vi "killApplication.vi"(8 "error in (no error)":errorcluster, 11 "VGS_RemoteControlClient in":refnum<class "VGS_RemoteControlClient.lvclass">) -> (0 "error out":errorcluster, 3 "VGS_RemoteControlClient out":refnum<class "VGS_RemoteControlClient.lvclass">)   [LabVIEW 2022 SP3, in "LV_VGS.lvlib" / "VGS_RemoteControlClient.lvclass"]
doc: "<B>Kills an existing VGStudio (MAX) instance. </B>\n\nThis method kills a running VGStudio (MAX) instance process, using the respective RemoteHandle. The method is used to unconditionally cause an application instance process to exit.\n\nParameters\nhandle A valid handle to an application instance. \n\nEmit error RemoteControlServiceIsNotAvailableException if the remote control service doesn't run. \nEmit error GenericRemoteControlErrorException if an internal error occurs.\nEmit error InvalidRemoteHandleException if the remote handle is not valid."
uses:
  VGS_RemoteControlClient.lvclass
  VGS_RemoteControlClient.lvclass/VGS_RemoteControlClient.ctl
  C:/Users/Andrey/Desktop/hajo/LV_VGS/vgs_project.dll
  vgs_project.dll
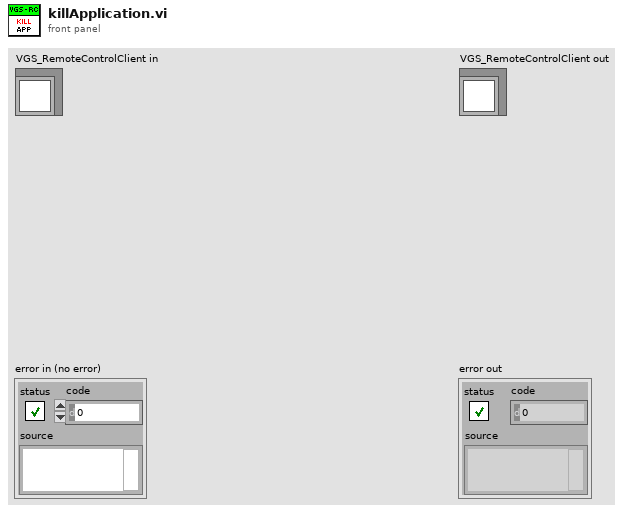
[diagram p1: front panel]
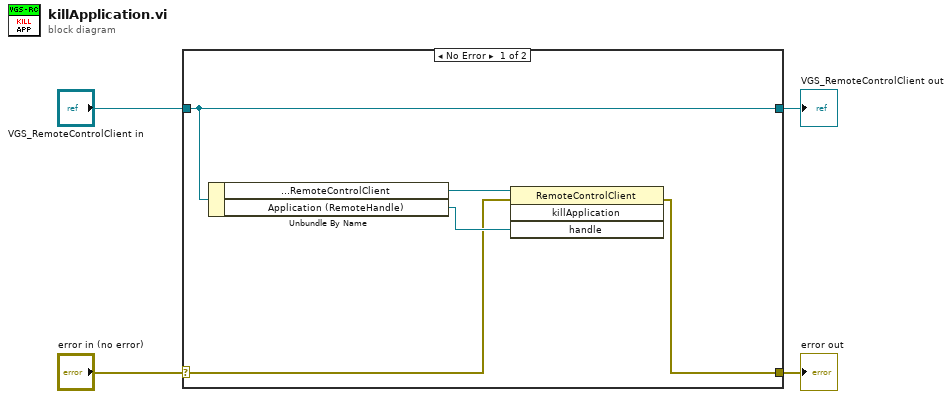
[diagram p0: block diagram]
diagram:
  n1 = case shown="No Error" "error in (no error)" {
    selector: "error in (no error)" -> [w6 w11]
    tunnel: [w5 w11] -> w3
    tunnel: [w9 w10] -> w1
    tunnel: "VGS_RemoteControlClient in" -> [w9 w10]
    frame No Error {
      n2 = Unbundle By Name(w9) -> ("VGS.Project.Interop.RemoteControlClient"=w8:refnum<k24>, "Application (RemoteHandle)"=w7:refnum<k24>)
      n3 = invoke class="RemoteControlClient" method="killApplication"(reference=w8, error in=w6, "handle"=w7) -> (error out=w5:errorcluster)  [unwired: 1 in, 3 out]
    }
    frame Error {
    }
  }
  "error out" <- w3
  "VGS_RemoteControlClient out" <- w1
